vi "ParserRegister.vi"(8 "error in (no error)":errorcluster, 11 "JSON item":string) -> (0 "error out":errorcluster, 2 "registers":T1[](array[typedef]), 3 "JSON item":string)   [LabVIEW 2017, in "Paser.lvlib"]
uses:
  Paser.lvlib
  <vilib>/JDP Science/JSONtext/JSONtext.lvlib
  Ctrl/Bitfield.ctl
  Ctrl/Register.ctl
  902fddd5-18d7-442a-9347-0e9ff130fe7a.vi
  fda50495-96e7-4f19-a4ce-27421a261046.vi
  6efc3bda-f626-426e-9550-7b00ef82c610.vi
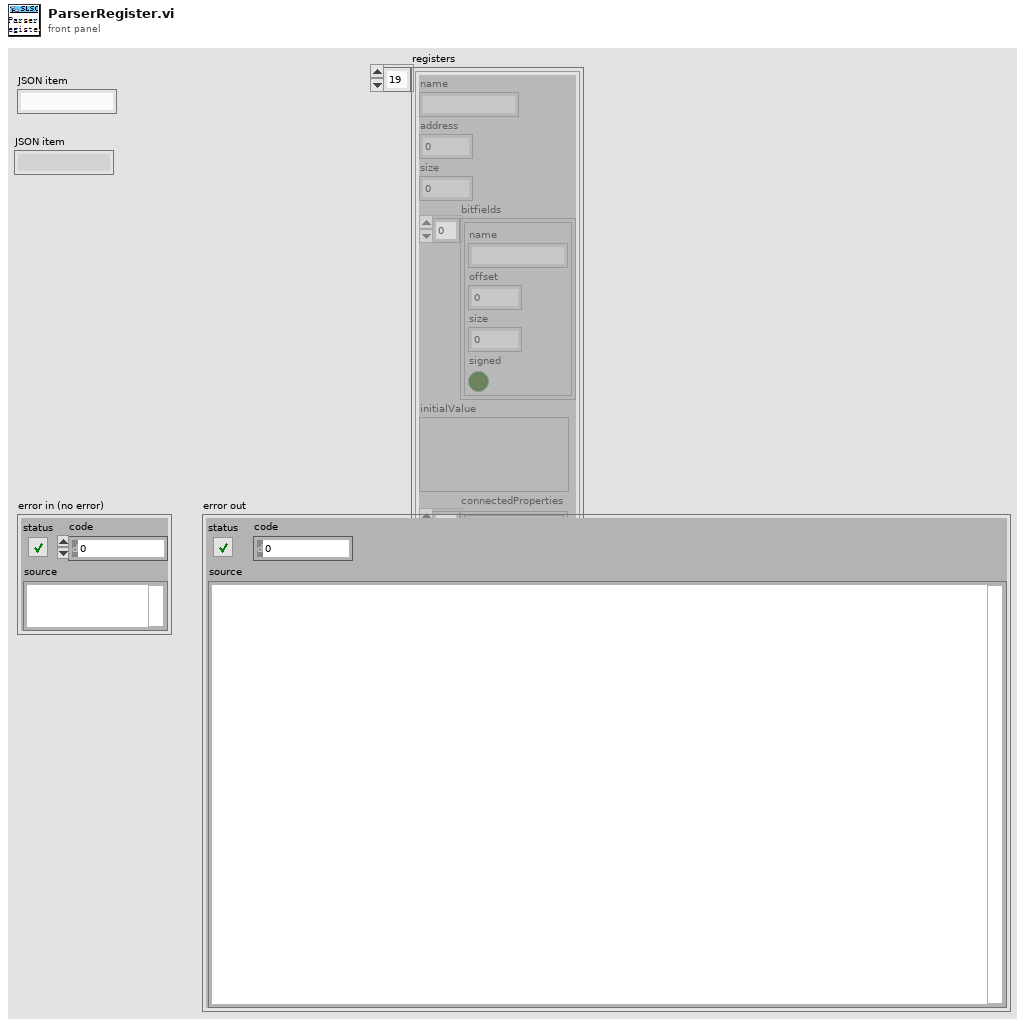
[diagram p1: front panel]
types:
  T1 = typedef "Register.ctl" = cluster{"name":string, "address":i32, "size":i32, "bitfields":T2[], "initialValue":variant, "connectedProperties":string[]}
  T2 = typedef "Bitfield.ctl" = cluster{"name":string, "offset":i32, "size":i32, "signed":bool}
  T3 = typedef "JSONtext.lvlib/JSON Value Type.ctl" = enum16{"Not a JSON Value", "JSON Object", "JSON Array", "String", "Number", "true", "false", "null"}
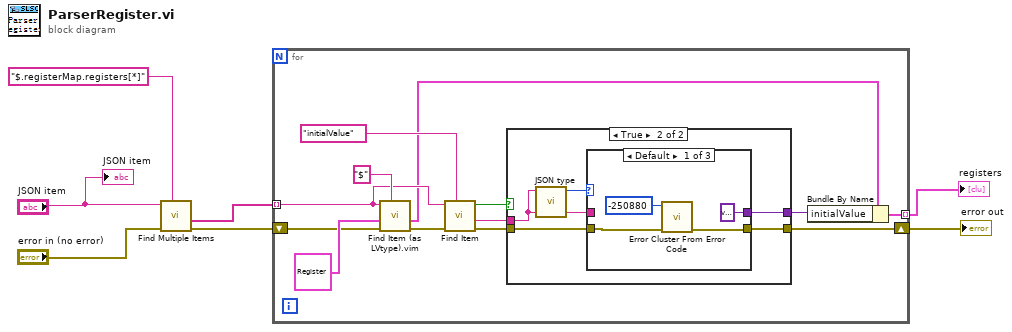
[diagram p0: block diagram]
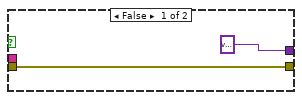
[diagram p2: hidden frame]
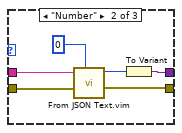
[diagram p3: hidden frame]
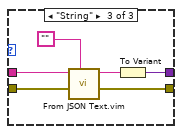
[diagram p4: hidden frame]
diagram:
  n1 = call <vilib>:"Find Multiple Items.vi"("$Path or Item Name"="$.registerMap.registers[*]", "error in (no error)"="error in (no error)", "JSON"="JSON item") -> ("error out"=w5:errorcluster, "<JSON>"=w4:string[])  [unwired: 5 in, 2 out]
  n2 = for {
    tunnel: w4 -> [w15] mode=indexing
    shift-right: [w11] -> w6
    shift-left: w5 -> [w19]
    tunnel: [w8] -> w7 mode=indexing
    n3 = call "Find Item (as LVtype).vim"("$Path or Item Name"="$", "error in (no error)"=w19, "Data Type and Default Value"=T1 {"name"="", "address"=0, "size"=0, "bitfields"=[], "initialValue"=variant, "connectedProperties"=[]}, "JSON"=w15) -> ("error out"=w17:errorcluster, "Data"=w10:T1)  [unwired: 4 in, 2 out]
    n4 = call <vilib>:"Find Item.vi"("$Path or Item Name"="initialValue", "error in (no error)"=w17, "JSON"=w15) -> ("error out"=w12:errorcluster, "<JSON>"=w14:string, "Found"=w13:bool)  [unwired: 5 in, 1 out]
    n5 = case shown="True" w13 {
      tunnel: w14 -> [_ w26]
      tunnel: w12 -> [w22 w25]
      tunnel: [w22 w24] -> w11
      tunnel: [variant w23] -> w9
      frame False {
      }
      frame True {
        n6 = call <vilib>:"JSON type.vi"("JSON"=w26) -> ("JSON Value Type"=w27:T3)  [unwired: 9 in, 1 out]
        n7 = case shown="Default" w27 {
          tunnel: w26 -> [_ w35 w43]
          tunnel: w25 -> [w31 w37 w41]
          tunnel: [w30 w36 w40] -> w24
          tunnel: [variant ("Variant") w32 w39] -> w23
          frame Default {
            n8 = call <vilib>:"Error Cluster From Error Code.vi"("error in (no error)"=w31, "error code (0)"=-250880) -> ("error out"=w30:errorcluster)  [unwired: 7 in]
          }
          frame "Number" {
            n9 = call "From JSON Text.vim"("Data Type and Default Value"=u64 0, "error in (no error)"=w37, "JSON"=w35) -> ("error out"=w36:errorcluster, "Data out"=w33:u64)  [unwired: 7 in]
            n10 = To Variant(anything=w33) -> (Variant=w32:variant)
          }
          frame "String" {
            n11 = call "From JSON Text.vim"("Data Type and Default Value"="" ("$Path or Item Name"), "error in (no error)"=w41, "JSON"=w43) -> ("error out"=w40:errorcluster, "Data out"=w38:string)  [unwired: 7 in]
            n12 = To Variant(anything=w38) -> (Variant=w39:variant)
          }
        }
      }
    }
    n13 = Bundle By Name(cluster=w10, "initialValue"=w9) -> (w8:T1)
  }
  "registers" <- w7
  "error out" <- w6
  "JSON item" <- "JSON item"
